vi "Test Deserialize.vi"(8 "error in (no error)":errorcluster) -> (0 "error out":errorcluster)   [LabVIEW 2017]
uses:
  <vilib>/addons/_JKI Toolkits/Caraya/classes/Test/Test.lvclass
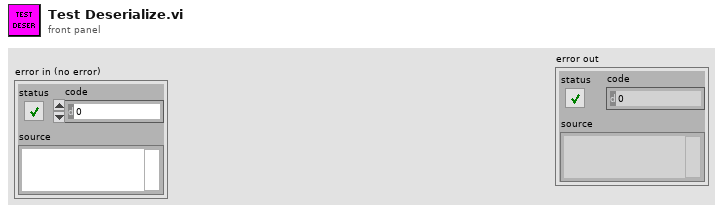
[diagram p1: front panel]
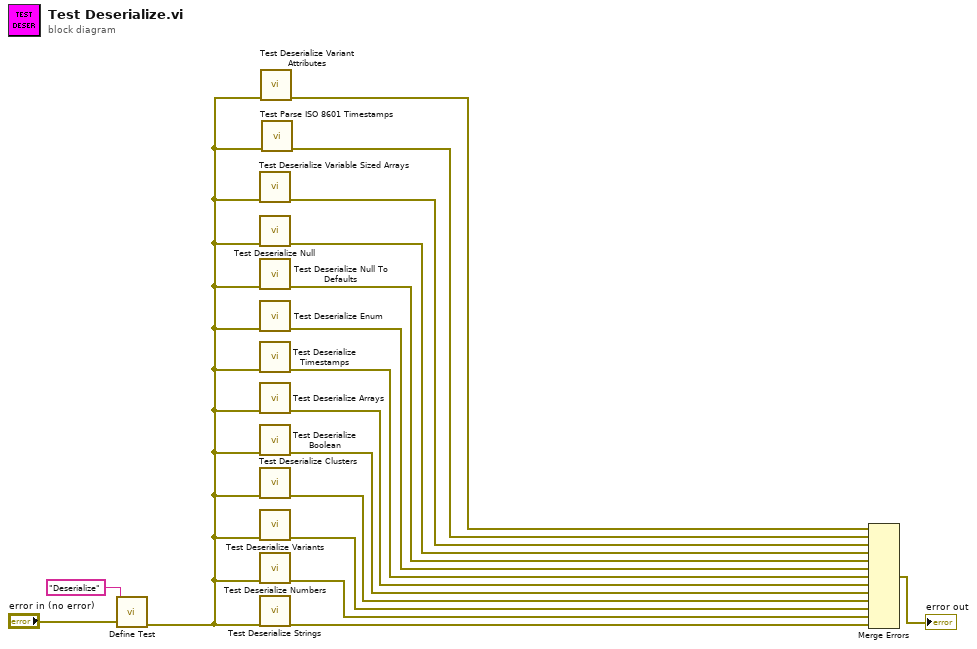
[diagram p0: block diagram]
diagram:
  n1 = call <vilib>:"Define Test.vi"("error in (no error)"="error in (no error)", "Label (VI Title)"="Deserialize") -> ("error out"=w2:errorcluster)  [unwired: 9 in]
  n2 = call "Test Deserialize Variable Sized Arrays.vi"("error in (no error)"=w2) -> ("error out"=w4:errorcluster)  [unwired: 10 in]
  n3 = call "Test Deserialize Null.vi"("error in (no error)"=w2) -> ("error out"=w5:errorcluster)  [unwired: 10 in]
  n4 = call "Test Deserialize Null To Defaults.vi"("error in (no error)"=w2) -> ("error out"=w6:errorcluster)  [unwired: 10 in]
  n5 = call "Test Deserialize Enum.vi"("error in (no error)"=w2) -> ("error out"=w7:errorcluster)  [unwired: 10 in]
  n6 = call "Test Deserialize Timestamps.vi"("error in (no error)"=w2) -> ("error out"=w8:errorcluster)  [unwired: 10 in]
  n7 = call "Test Deserialize Arrays.vi"("error in (no error)"=w2) -> ("error out"=w9:errorcluster)  [unwired: 10 in]
  n8 = call "Test Deserialize Boolean.vi"("error in (no error)"=w2) -> ("error out"=w10:errorcluster)  [unwired: 10 in]
  n9 = call "Test Deserialize Clusters.vi"("error in (no error)"=w2) -> ("error out"=w11:errorcluster)  [unwired: 10 in]
  n10 = call "Test Deserialize Variants.vi"("error in (no error)"=w2) -> ("error out"=w12:errorcluster)  [unwired: 10 in]
  n11 = call "Test Deserialize Numbers.vi"("error in (no error)"=w2) -> ("error out"=w13:errorcluster)  [unwired: 10 in]
  n12 = call "Test Deserialize Strings.vi"("error in (no error)"=w2) -> ("error out"=w14:errorcluster)  [unwired: 10 in]
  n13 = call "Test Deserialize Variant Attributes.vi"("error in (no error)"=w2) -> ("error out"=w1:errorcluster)  [unwired: 10 in]
  n14 = call "Test Parse ISO 8601 Timestamps.vi"("error in (no error)"=w2) -> ("error out"=w3:errorcluster)  [unwired: 10 in]
  n15 = Merge Errors(w1, w3, w4, w5, w6, w7, w8, w9, w10, w11, w12, w13, w14) -> (→"error out":errorcluster)
